vi "Lossy Stream.vi"() -> ()   [LabVIEW 2023]
doc: "This VI demonstrates the behavior of the Lossy Stream, a channel wire that communicates data between two parallel loops but never blocks the writer -- when the buffer gets full, it simply drops data."
uses:
  <vilib>/ChannelSupport/Lossy Behavior.ctl
  <extravilib>/ChannelInstances/Lossy Stream-dbl/Write With Abort.vi
  <extravilib>/ChannelInstances/Lossy Stream-dbl/Read With Abort.vi
  <extravilib>/ChannelInstances/Lossy Stream-dbl/Endpoint.vi
  <extravilib>/ChannelInstances/Lossy Stream-dbl/EndpointRead.vi
  <extravilib>/ChannelInstances/Lossy Stream-dbl/Instantiate.vi
  <extravilib>/ChannelInstances/Lossy Stream-dbl/)Channel.vi
  <resource>/ChannelSupport/_ChannelSupport/WaitIfNeeded.vi
  <extravilib>/ChannelInstances/Lossy Stream-dbl.lvlib
panel:
  out "Data lost":bool
  in  "lossy behavior":T1
  out "Gap":bool
  out "Level":dbl(slide) scale=0.0..1.0
  out "Data Consumed":dbl(graph)
  out "Data Produced":dbl(graph)
  in  "Stall":bool
  in  "Stop":bool
  # "Overview: Demonstrates the Lossy Stream channel. Lossy Streams are restricted to a single writer and a single reader to provide point-to-point communication. The Lossy Stream behaves like a Stream except that it never blocks the writer: when the Lossy Stream is full, it simply drops data when another write is attempted. The Lossy Stream can be configured to drop either the oldest data or the newest data, and in either case the reader can detect when data was dropped. \n\nInstructions:\n1. Run the VI. Observe the producer and the consumer showing the same continuous data.\n2. Press and hold the Stall Consumer button to see the Lossy Stream fill up and lose data.\n3. Release the Stall Consumer button and notice the flash of the Gap indicator as well as the discontinuity in the Data Consumed graph. If behavior is drop oldest Gap will flash immediately after releasing Stall, otherwise there will be a slight delay as the buffer empties the old data after which the gap will appear."
  # "Set This Before Running VI"
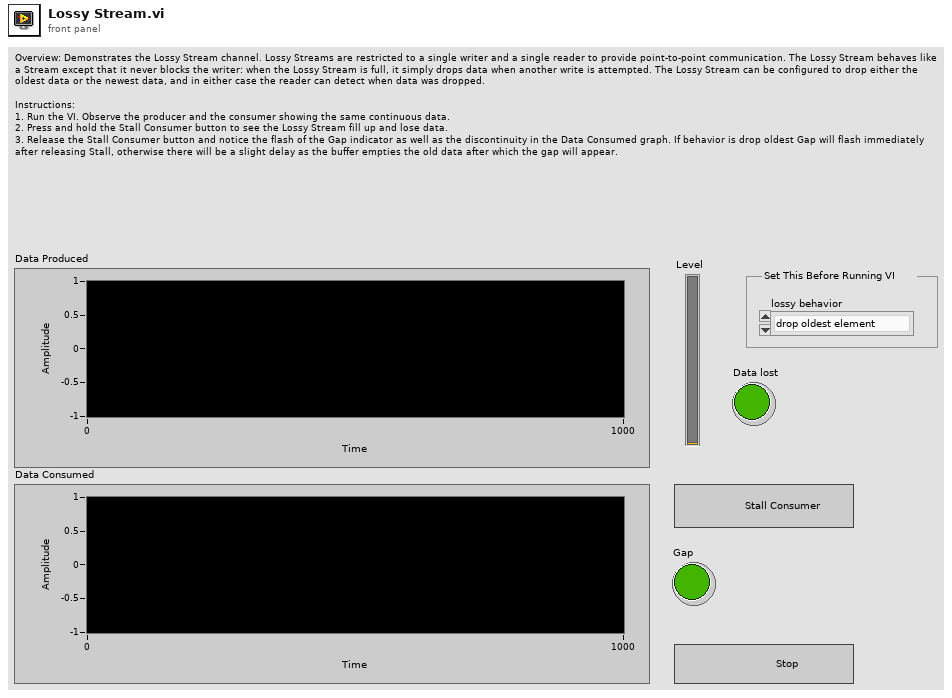
[diagram p1: front panel]
types:
  T1 = typedef "Lossy Behavior.ctl" = enum16{"drop oldest element", "skip this write"}
  T2 = typedef "Lossy Stream-dbl.lvlib/)Channel.ctl" = refnum<queue>
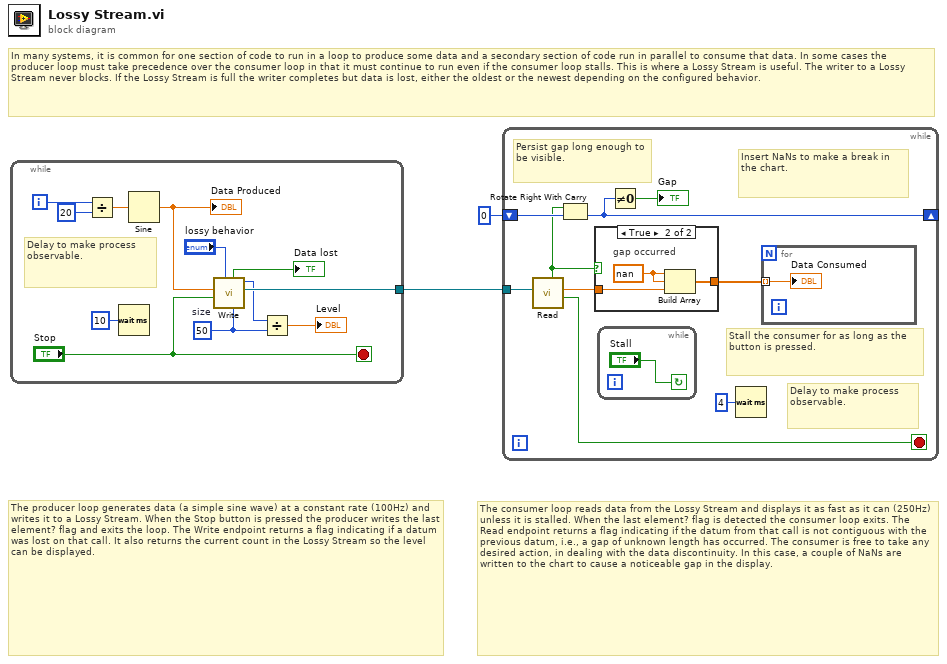
[diagram p0: block diagram]
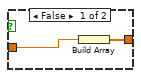
[diagram p2: hidden frame]
diagram:
  # "The consumer loop reads data from the Lossy Stream and displays it as fast as it can (250Hz) unless it is stalled. When the last element? flag is detected the consumer loop exits. The Read endpoint returns a flag indicating if the datum from that call is not contiguous with the previous datum, i.e., a gap of unknown length has occurred. The consumer is free to take any desired action, in dealing with the data discontinuity. In this case, a couple of NaNs are written to the chart to cause a noticeable gap in the display."
  # "The producer loop generates data (a simple sine wave) at a constant rate (100Hz) and writes it to a Lossy Stream. When the Stop button is pressed the producer writes the last element? flag and exits the loop. The Write endpoint returns a flag indicating if a datum was lost on that call. It also returns the current count in the Lossy Stream so the level can be displayed."
  # "In many systems, it is common for one section of code to run in a loop to produce some data and a secondary section of code run in parallel to consume that data. In some cases the producer loop must take precedence over the consumer loop in that it must continue to run even if the consumer loop stalls. This is where a Lossy Stream is useful. The writer to a Lossy Stream never blocks. If the Lossy Stream is full the writer completes but data is lost, either the oldest or the newest depending on the configured behavior."
  n1 = while {
    tunnel: [w9] -> w2
    i -> [w14]
    stop <- "Stop" stop-if-true
    w7 = 50  # size
    # "Delay to make process observable."
    n2 = Divide(x=w14, y=20) -> (x/y=w12:dbl)
    n3 = Wait (ms)(milliseconds to wait=u32 10) -> ()  [unwired: 1 out]
    n4 = Sine(x=w12) -> (sin(x)=w11:dbl)
    "Data Produced" <- w11
    n5 = call <extravilib>:"Write.vi"("size (1)"=w7, "lossy behavior (drop oldest)"="lossy behavior", "last element? (F)"="Stop", "element"=w11) -> ("channel"=w9:T2, "count"=w6:i32, "data lost?"=→"Data lost":bool)  [unwired: 5 in]
    n6 = Divide(x=w6, y=w7) -> (x/y=→"Level":dbl)
  }
  n7 = while {
    tunnel: w2 -> [w23]
    shift-right: [w18] -> _
    shift-left: u16 0 -> [w19]
    stop <- w22 stop-if-true
    # "Stall the consumer for as long as the button is pressed."
    # "Insert NaNs to make a break in the chart."
    # "Persist gap long enough to be visible."
    # "Delay to make process observable."
    n8 = call <extravilib>:"Read.vi"("channel"=w23) -> ("last element?"=w22:bool, "element"=w21:dbl, "gap?"=w16:bool)  [unwired: 5 in, 3 out]
    n9 = Rotate Right With Carry(2:w19, 3:w16) -> (0:w18:u16)  [unwired: 1 out]
    n10 = case shown="True" w16 {
      tunnel: w21 -> [w26 w29]
      tunnel: [w25 w28] -> w20
      frame False {
        n11 = Build Array(w26) -> (w25:dbl[])
      }
      frame True {
        w27 = nan
        # "gap occurred"
        n12 = Build Array(w27, w27, w29) -> (w28:dbl[])
      }
    }
    n13 = while {
      stop <- "Stall" continue-if-true
    }
    n14 = Not Equal To 0?(x=w18) -> (x != 0?=→"Gap":bool)
    n15 = Wait (ms)(milliseconds to wait=u32 4) -> ()  [unwired: 1 out]
    n16 = for {
      tunnel: w20 -> [w24] mode=indexing
      "Data Consumed" <- w24
    }
  }
